vi "main 0.6.vi"() -> ()   [LabVIEW 2015]
uses:
  subvi/PHOIBOS/DEFINITIONS/DEF_dev_state.ctl
  subvi/PHOIBOS/DEFINITIONS/DEF_dev_type.ctl
  <vilib>/Utility/file.llb/Write Delimited Spreadsheet (DBL).vi
  subvi/Newport ESP301/Newport ESP301.lvlib
  subvi/sp_manip.llb/sp_manip_lib.lvlib
  subvi/sp_manip.llb/tcp_gateway.lvlib
panel:
  out "RunNumber":u16=4
  out "# elements in queue":i32
  out "sum":dbl=3886353.0
  out "cam_fps":dbl(slide)=19.67681433793903 caption="FPS" scale=0.1..50.0
  out "max value":u32=54
  out "Intensity Graph":dbl[][](graph)
  out "ESP_con?":bool=TRUE caption="ESP301"
  out "phoib_con?":bool caption="PHOIBOS"
  out "manip_con?":bool caption="manipulator"
  out "cam_con?":bool caption="camera"
  in  "main_close":bool
  in  "Tab Control":T1(tab)
  in  "cam_avg":u32=20
  in  "ESP_delta":dbl caption="relative [mm]"
  in  "ESP_-":bool
  in  "ESP_+":bool
  in  "ESP_go":bool
  in  "ESP_dest_t":dbl caption="Delay [fs]"
  in  "ESP_dest":dbl=33.3075 caption="Position [mm]"
  in  "ESP_set_t0":bool
  in  "phoib_I_6s":dbl=3200.0
  in  "phoib_I_5s":dbl=1400.0
  in  "phoib_I_4s":dbl=4.2
  in  "phoib_I_3s":dbl
  in  "phoib_I_2s":dbl=35.0
  in  "phoib_I_1s":dbl=21.9
  in  "phoib_standby":bool
  in  "phoib_set":bool
  out "phoib_I_6":dbl caption="Screen Voltage"
  out "phoib_I_5":dbl caption="Detctor Voltage"
  out "phoib_I_4":dbl caption="Work Function"
  out "phoib_I_3":dbl caption="Coil Current"
  out "phoib_I_2":dbl caption="Pass Energy"
  out "phoib_I_1":dbl caption="Kinetic Energy"
  out "Saved Positions":string[][](table)=[["ertwertwert", "-2.299945", "-2.030214", "38.900024", "50.000762", "0.000887", "-97.998082"], ["uztgugt", "-14.999451", "-13.638894", "442.380066", "13.998380", "-1.893758", "-76.305838"], ["asdf", "-14.999451", "-13.638894", "442.380066", "13.998380", "-1.893758", "-76.305838"], ["test3", "-14.999451", "-13.638894", "441.380066", "13.998380", "-1.893758", "-76.305838"]]
  in  "Save Pos":bool
  in  "Load":bool
  in  "Delete":bool
  in  "ManipRel":dbl=1.0
  in  "ManipRel +":bool
  in  "ManipRel -":bool
  in  "manip.rel.select":enum32{"x", "y", "z", "polar", "tilt", "azimut"}(radio)=enum."polar"
  in  "Move Abs":bool
  in  "stop manip":bool
  in  "dest":dbl[](array[numeric])=[0.007141549166819264, -0.009888298846365134, 431.30615234375, 89.00040512814502, 1.109125024699864, -227.9162918846475] caption="destinations" format="%#.5g"
  out "names":string[](array[string])=["x", "y", "z", "polar", "tilt", "azimut"]
  out "pos":dbl[](array[numeric])=[0.007141549166819264, -0.009888298846365134, 431.30615234375, 89.00040512814502, 1.109125024699864, -227.9162918846475] caption="positions" format="%.5f"
  in  "Mode":T2(ring)=enum."WideAngleMode"
  in  "VoltageRange":enum16{"3.5kV", "1.5kV", "400V", "100V", "10V"}(ring)=enum."400V"
  out "ESP_pos":dbl=33.3075 caption="Position"
  out "ESP_delay":dbl caption="Delay"
  out "ESP_t0":dbl=33.3075 caption="Time Zero @"
  out "phoib_I_7":dbl caption="Conversion Voltage"
  in  "phoib_I_7s":dbl
  in  "phoib_I_8s":dbl
  in  "phoib_I_9s":dbl
  out "phoib_I_8":dbl caption="FD1"
  out "phoib_I_9":dbl caption="FD2"
  out "electronics temp [°C]":i32=30
  out "CCD temp [°C]":i32=-13
  in  "gain":bool
  in  "exposure [ms]":u32=20
  in  "binning":u16(ring)=2 items=["X 1", "X 2", "X 4", "X 8"]
  in  "cam_dark?":bool caption="subtract dark?"
  in  "cam_dark":bool
  in  "cam_dark#":u32 max=1000
  in  "cam_burst":bool
  in  "cam_burstnr":u32 max=100000
  out "cam_burst_progress":i32(slide) scale=0.0..10.0
  out "Motion Done":bool
  in  "delscan_picspstep":u16=1 caption="pics/step" min=1 step=1
  in  "delscan_abort":bool
  out "delscan_progress":u32(slide) scale=0.0..20.0
  in  "delscan_go":bool
  out "delscan_pos":dbl caption="current delay [fs]"
  in  "delscan_end":dbl caption="end [fs]"
  in  "delscan_stepsize":dbl caption="stepsize [fs]"
  in  "delscan_start":dbl caption="start [fs]"
  in  "comment":string
  out "opti_frames":dbl=25.0 caption="#steps_opti"
  out "opti_current_frame":i32=25
  out "Measurement Progress":u8(slide) scale=0.0..100.0
  out "Camera Aquisition":u8(slide) scale=0.0..100.0
  in  "Optimize":bool
  in  "OptiStepSize":dbl=-1.0 caption="Step Size"
  in  "OptiRange":dbl=25.0 caption="Range"
  in  "meas_axis":string(combo)="tilt" caption="Axis"
  in  "meas_avg":i32=60 caption="Frames2Average"
  in  "OptiCancel":bool
  out "#steps_opti":dbl=25.0
  out "current_step_opti":i32=25
  out "ETA":string
  in  "BasePath":path=path "Z:/PESdata"
  in  "Path":path=path "Z:/software/ManipulatorControl/save.txt"
  in  "ROI Bottom":i32=32
  in  "ROI Top":i32=1
  in  "ROI Right":i32=40
  in  "ROI Left":i32=1
  in  "ESP Axis":i32=1 min=1 max=3
  in  "manip_init":bool
  in  "manip_release":bool
  in  "phoib_init":bool
  in  "phoib_release":bool
  in  "ESP_init":bool
  in  "ESP_release":bool
  in  "ESP301 VISA":refnum<visa-resource-name>="COM8"
  in  "cam_boardnr":i32
  in  "cam_init":bool
  in  "cam_release":bool
  out "error out":errorcluster
  out "error out 2":errorcluster
  out "state":T3 items=["Off"=-1, "Standby"=0, "On"=1]
  # "step _ of _"
  # "step _ of _"
  # "manip"
  # "phoib"
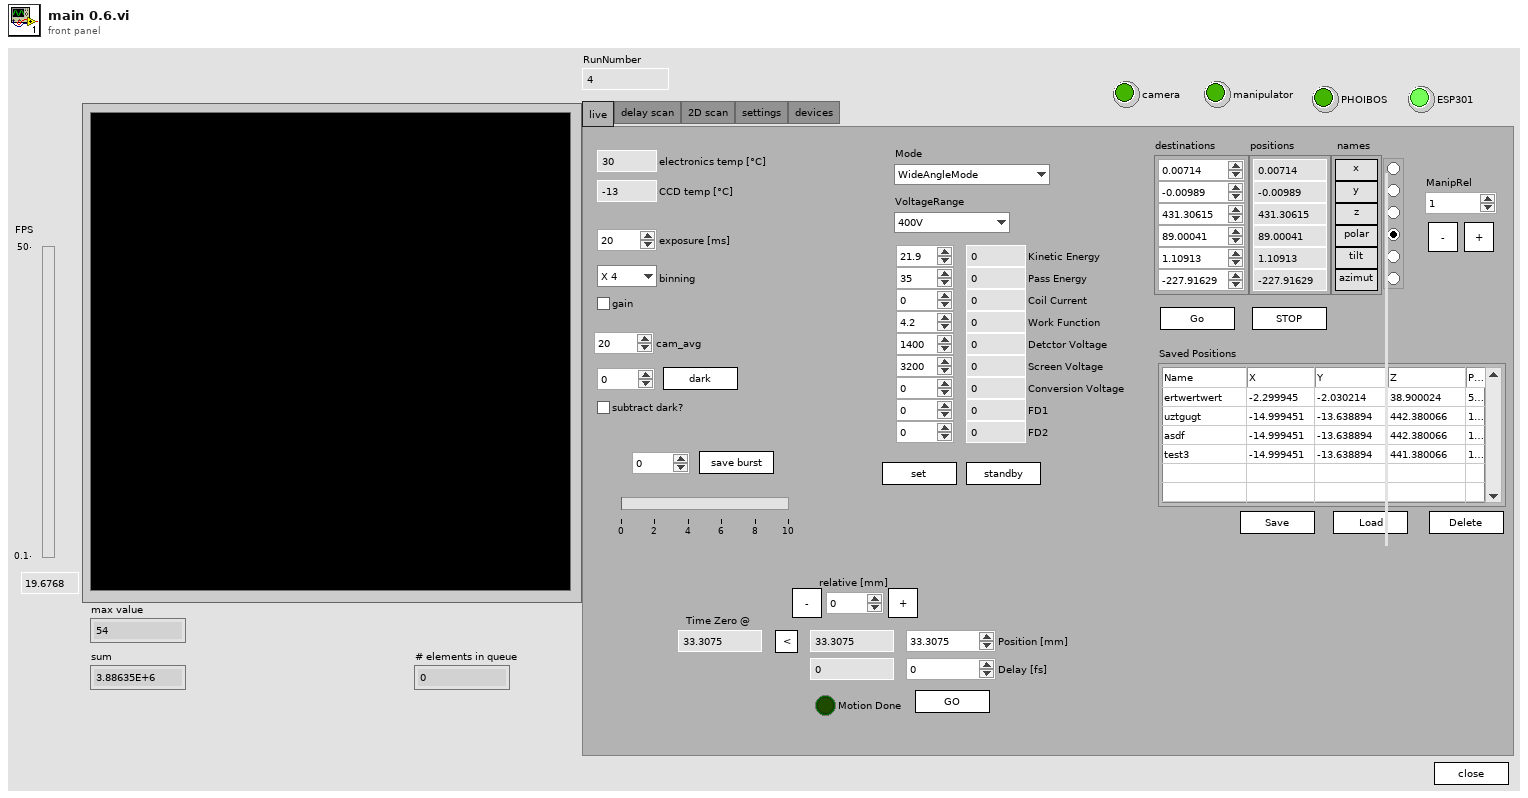
[diagram p1: front panel]
types:
  T1 = enum32{"live", "delay scan", "2D scan", "settings", "devices"}
  T2 = enum16{"HighMagnification", "MediumMagnification", "LowMagnification", "HighAngularDispersion", "MediumAngularDispersion", "LowAngularDispersion", "WideAngleMode", "LargeArea", "MediumArea", "SmallArea", "HighMagnification2", "SmallArea2", "ImagingMode"}
  T3 = typedef "DEF_dev_state.ctl" = i32
  T4 = enum16{"open", "replace", "create", "open or create", "replace or create", "replace or create with confirmation"}
  T5 = cluster{"Camera type":u32, "Operating mode\nHP & QE / HS & DiCam Pro ":u32, "Frame trigger \n(High Performance and QE only)":u16, "Sequence trigger":u16, "Low Light\n(QE only)":bool, "Gain":bool, "Horzontal\nbinning":u16, "Vertical\nbinning ":u16, "ROI Left":i32, "ROI Right":i32, "ROI Top":i32, "ROI Bottom":i32}
  T6 = cluster{"Axis_Name":string, "Axis_Type":string, "Axis_Position":dbl, "continous":bool, "moving":bool}[]
  T7 = cluster{"Axis_Name":string, "Axis_Type":string, "Axis_Position":dbl, "continous":bool, "moving":bool}
  T8 = typedef "DEF_dev_type.ctl" = enum32{"devA (analyzer)", "devD (detector)"}
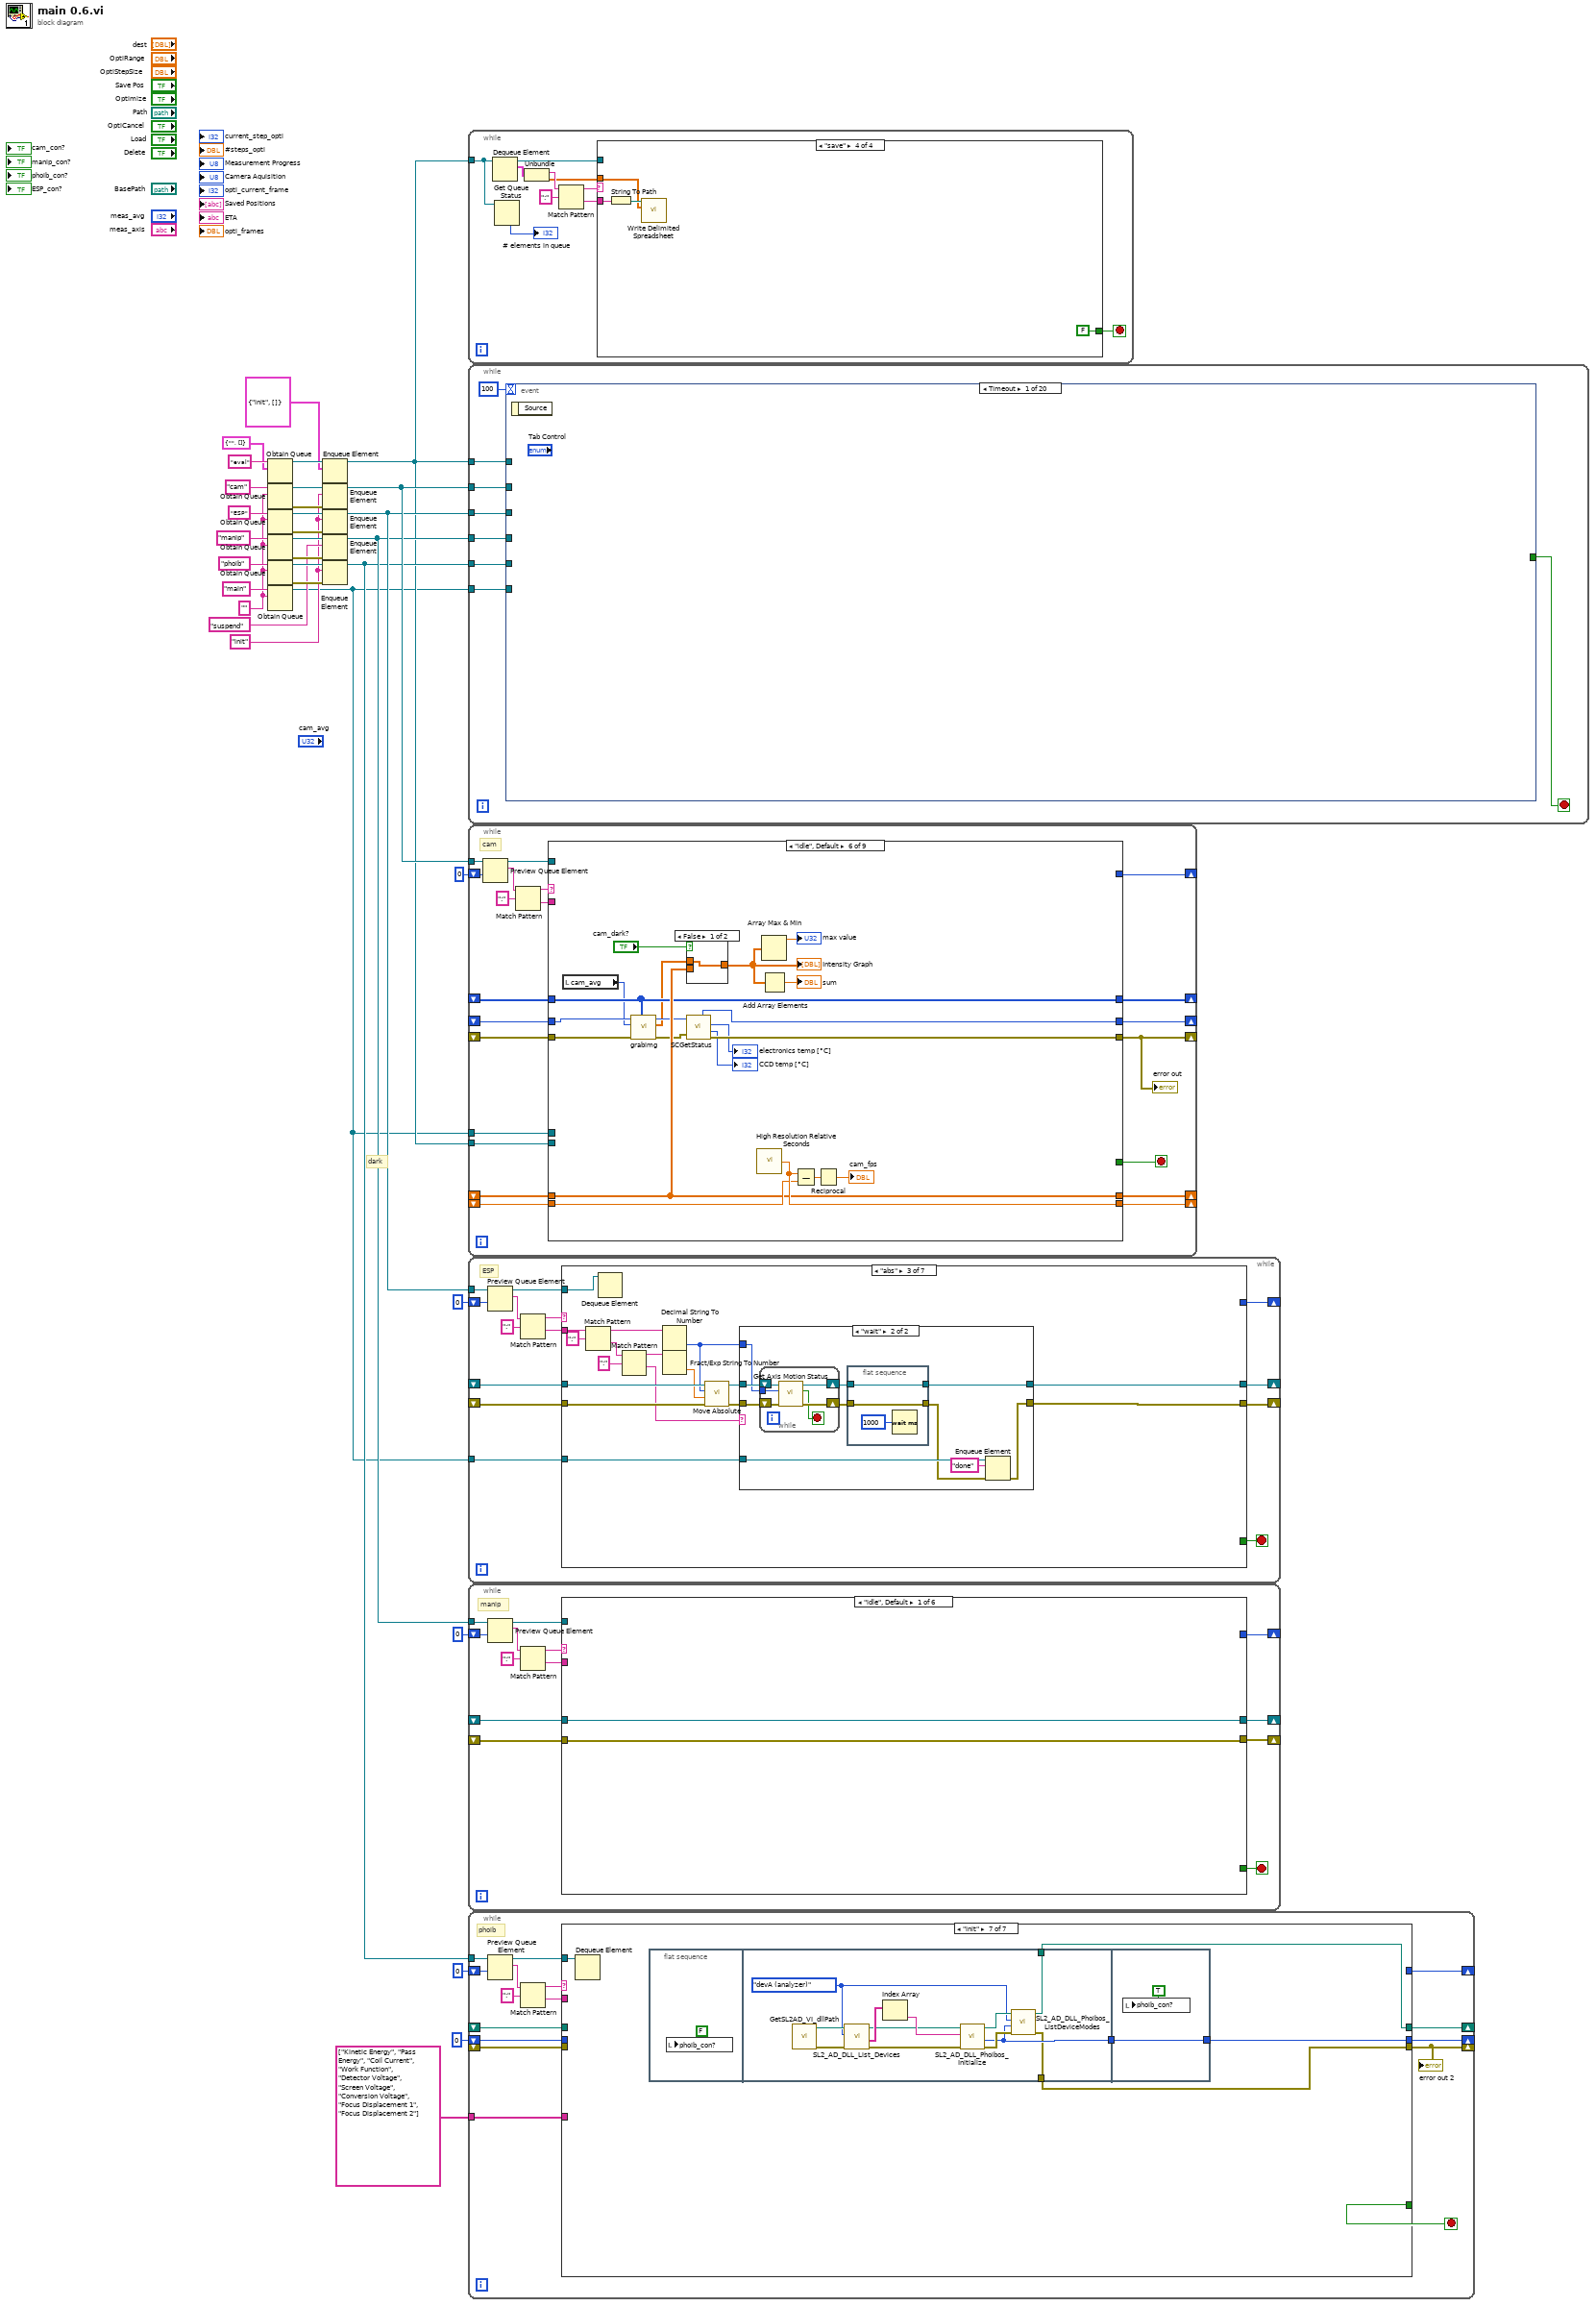
[diagram p0: block diagram]
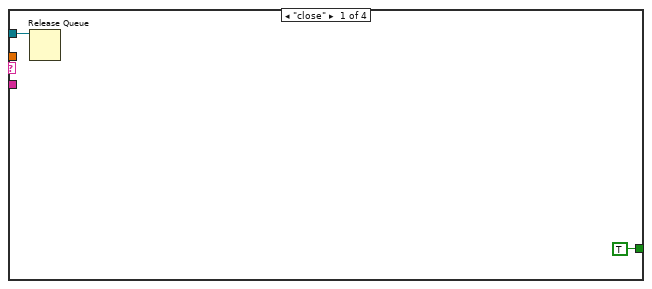
[diagram p2: hidden frame]
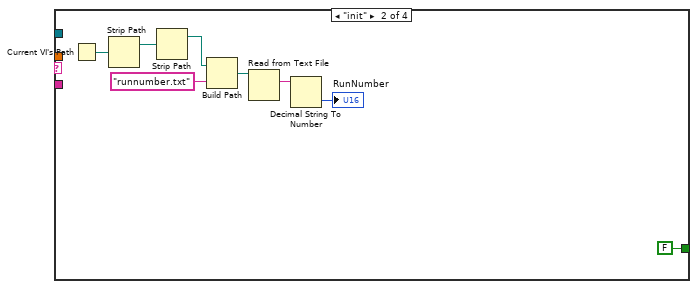
[diagram p3: hidden frame]
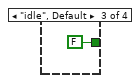
[diagram p4: hidden frame]
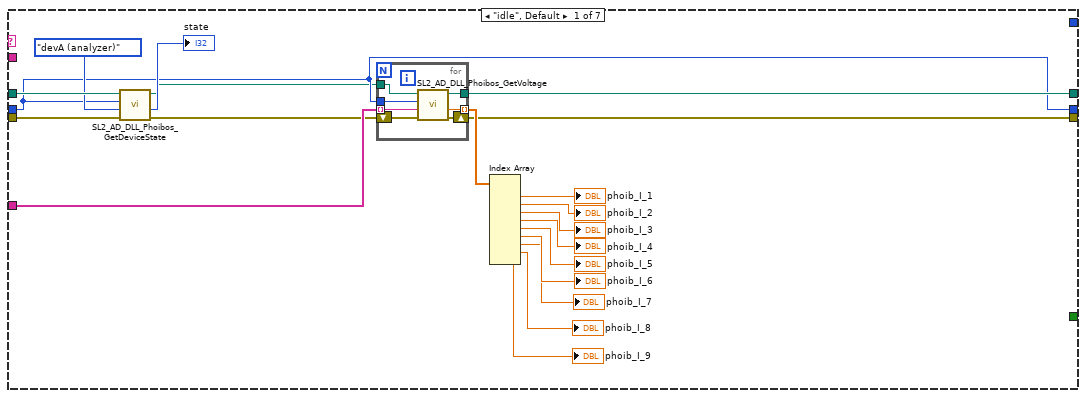
[diagram p5: hidden frame]
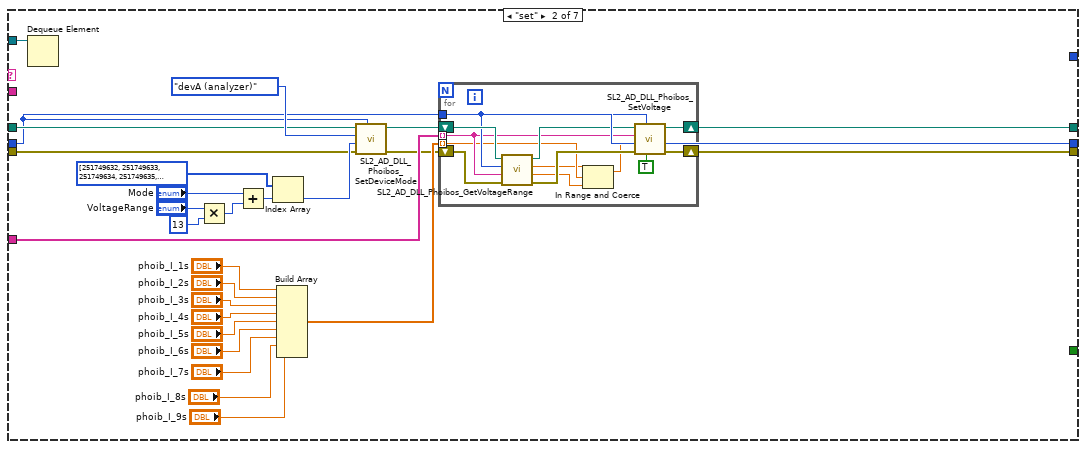
[diagram p6: hidden frame]
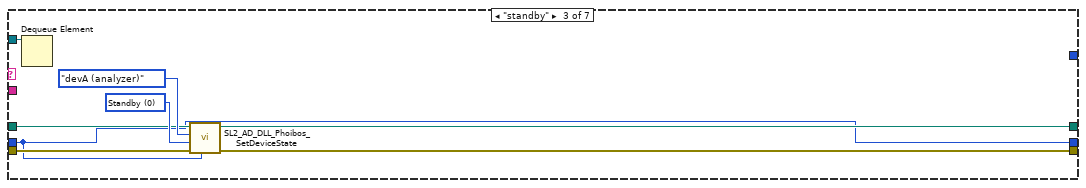
[diagram p7: hidden frame]
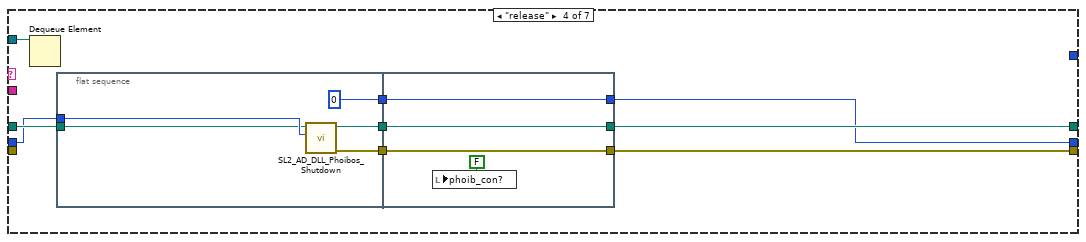
[diagram p8: hidden frame]
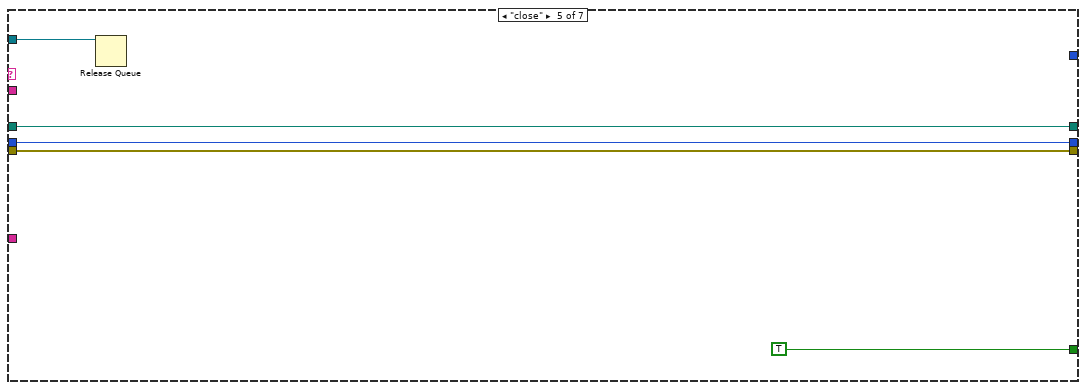
[diagram p9: hidden frame]
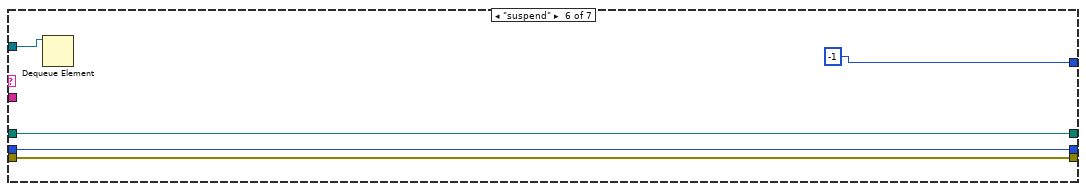
[diagram p10: hidden frame]
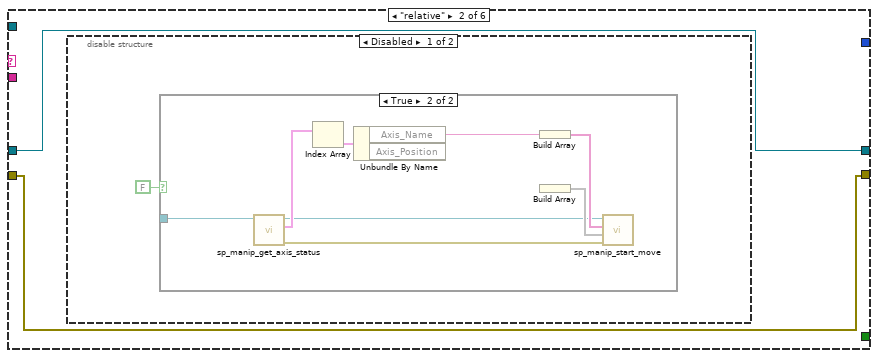
[diagram p11: hidden frame]
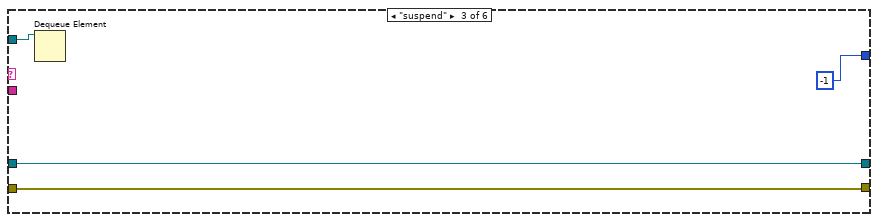
[diagram p14: hidden frame]
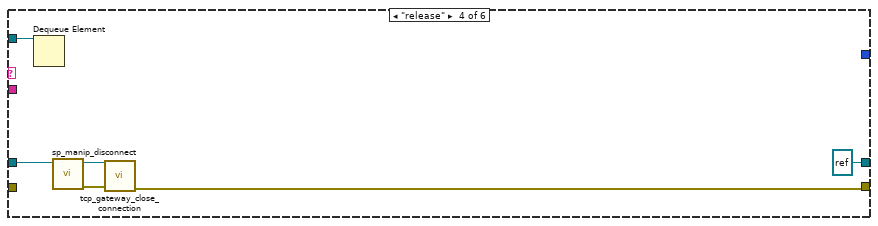
[diagram p15: hidden frame]
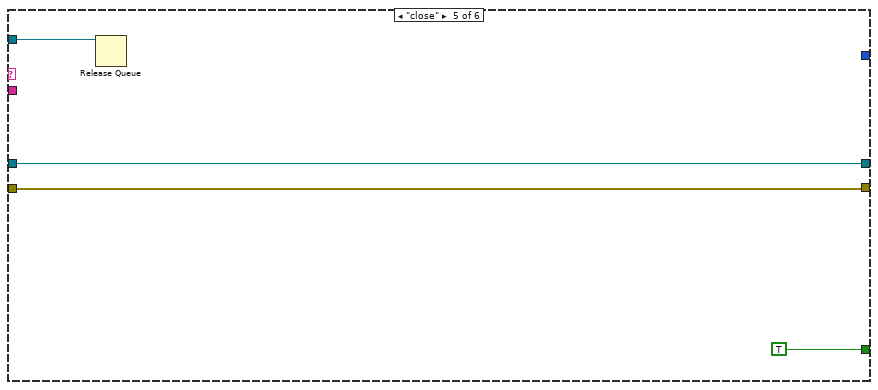
[diagram p16: hidden frame]
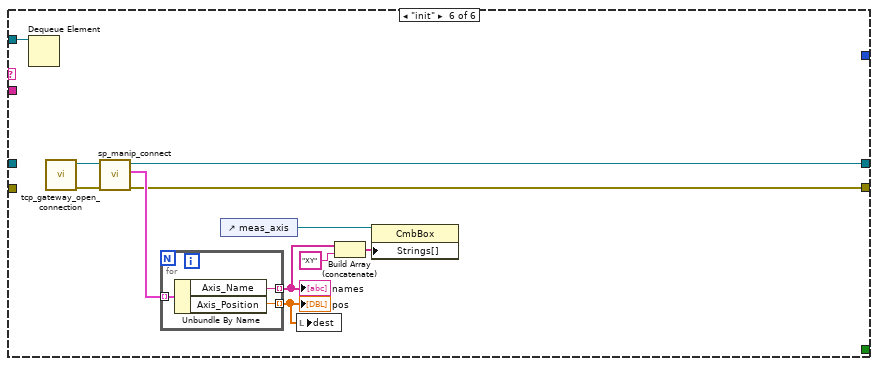
[diagram p17: hidden frame]
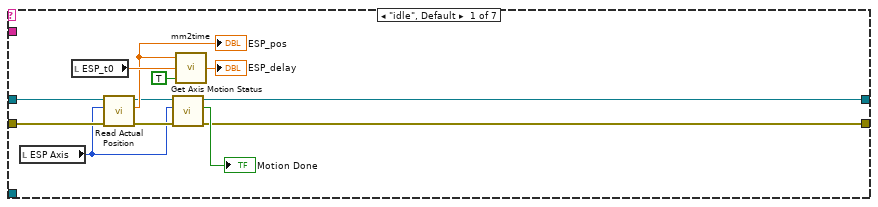
[diagram p18: hidden frame]
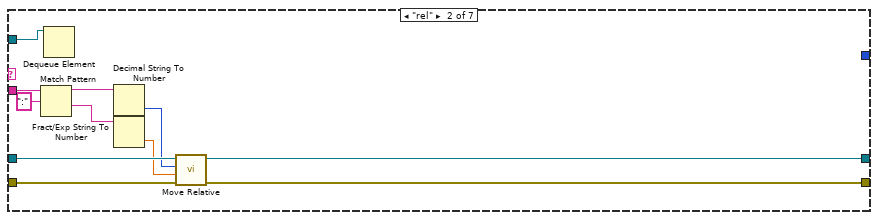
[diagram p19: hidden frame]
diagram:
  w3 = "init" ("name (unnamed)")
  w8 = "" ("name (unnamed)")
  # "dark"
  n1 = Obtain Queue(name (unnamed)="eval", element data type=cluster{string, dbl[][]} {"", []}) -> (queue out=w6:refnum<queue>)  [unwired: 3 in, 2 out]
  n2 = Obtain Queue(name (unnamed)="cam", element data type=w8) -> (queue out=w31:refnum<queue>, error out=w30:errorcluster)  [unwired: 3 in, 1 out]
  n3 = Obtain Queue(name (unnamed)="ESP", element data type=w8) -> (queue out=w27:refnum<queue>, error out=w28:errorcluster)  [unwired: 3 in, 1 out]
  n4 = Obtain Queue(name (unnamed)="manip", element data type=w8) -> (queue out=w24:refnum<queue>, error out=w23:errorcluster)  [unwired: 3 in, 1 out]
  n5 = Obtain Queue(name (unnamed)="phoib", element data type=w8) -> (queue out=w21:refnum<queue>, error out=w22:errorcluster)  [unwired: 3 in, 1 out]
  n6 = Obtain Queue(name (unnamed)="main", element data type=w8) -> (queue out=w1:refnum<queue>)  [unwired: 3 in, 2 out]
  n7 = Enqueue Element(queue=w6, element=cluster{string, dbl[][]} {"init", []}) -> (queue out=w5:refnum<queue>)  [unwired: 2 in, 2 out]
  n8 = Enqueue Element(queue=w31, element=w3, error in (no error)=w30) -> (queue out=w29:refnum<queue>)  [unwired: 1 in, 2 out]
  n9 = Enqueue Element(queue=w27, element=w3, error in (no error)=w28) -> (queue out=w18:refnum<queue>)  [unwired: 1 in, 2 out]
  n10 = Enqueue Element(queue=w24, element="suspend" ("name (unnamed)"), error in (no error)=w23) -> (queue out=w17:refnum<queue>)  [unwired: 1 in, 2 out]
  n11 = Enqueue Element(queue=w21, element=w3, error in (no error)=w22) -> (queue out=w16:refnum<queue>)  [unwired: 1 in, 2 out]
  n12 = while {
    tunnel: w5 -> [w34]
    stop <- w35 stop-if-true
    n13 = Dequeue Element(queue=w34) -> (queue out=w40:refnum<queue>, element=w39:cluster{string, dbl[][]})  [unwired: 2 in, 2 out]
    n14 = Get Queue Status(queue=w34) -> (# elements in queue=→"# elements in queue":i32)  [unwired: 2 in, 7 out]
    n15 = Unbundle(w39) -> (w38:string, w37:dbl[][])
    n16 = Match Pattern(string=w38, regular expression=":") -> (before substring=w41:string, after substring=w36:string)  [unwired: 1 in, 2 out]
    n17 = case shown="\"save\"" w41 {
      tunnel: w40 -> [w44 _ _ _]
      tunnel: w37 -> [_ _ _ w55]
      tunnel: w36 -> [_ _ _ w57]
      tunnel: [TRUE FALSE FALSE FALSE] -> w35
      frame "close" {
        n18 = Release Queue(queue=w44) -> ()  [unwired: 2 in, 3 out]
      }
      frame "init" {
        n19 = Current VI's Path() -> (path=w51:path)
        n20 = Strip Path(path=w51) -> (stripped path=w46:path)  [unwired: 1 out]
        n21 = Strip Path(path=w46) -> (stripped path=w45:path)  [unwired: 1 out]
        n22 = Build Path(base path=w45, name or relative path="runnumber.txt") -> (appended path=w49:path)
        n23 = Read from Text File(file (use dialog)=w49) -> (text=w48:string)  [unwired: 3 in, 3 out]
        n24 = Decimal String To Number(string=w48) -> (number=→"RunNumber":i32)  [unwired: 2 in, 1 out]
      }
      frame "idle", Default {
      }
      frame "save" {
        n25 = String To Path(string=w57) -> (path=w56:path)
        n26 = call-poly <vilib>:"Write Delimited Spreadsheet.vi"("file path (dialog if empty)"=w56, "2D data"=w55) -> ()  [unwired: 12 in, 2 out]
      }
    }
  }
  n27 = while {
    tunnel: w29 -> [w63]
    tunnel: w18 -> [w62]
    tunnel: w17 -> [w61]
    tunnel: w16 -> [w60]
    tunnel: w1 -> [w59]
    tunnel: w5 -> [w58]
    stop <- w65 stop-if-true
    n28 = event shown="[0] Timeout" {
      selector: _ -> [_ _ _ _ _ _ _ _ _ _ _ _ _ _ _ _ _ _ _ _]
      dyn-events: _ -> [_ _ _ _ _ _ _ _ _ _ _ _ _ _ _ _ _ _ _ _]
      timeout: 100 -> [_ _ _ _ _ _ _ _ _ _ _ _ _ _ _ _ _ _ _ _]
      tunnel: [_ TRUE _ _ _ _ _ _ _ _ _ _ _ _ _ _ _ _ _ _] -> w65
      tunnel: w63 -> [_ w78 w81 _ _ _ _ _ w107 w109 w110 _ _ _ _ _ _ _ _ w202]
      tunnel: w62 -> [_ w77 _ w85 _ _ _ _ _ _ _ _ _ _ w156 _ w168 _ _ w204]
      tunnel: w61 -> [_ w76 _ _ w91 _ _ _ _ _ _ _ _ _ _ _ _ _ _ _]
      tunnel: w60 -> [_ w75 _ _ _ w97 w103 w104 _ _ _ _ _ _ _ _ _ _ _ _]
      tunnel: w59 -> [_ w68 _ _ _ _ _ _ _ _ _ _ _ _ _ _ _ _ _ w203]
      tunnel: w58 -> [_ w67 _ _ _ _ _ _ _ _ _ _ _ _ _ _ _ _ _ _]
      event Timeout {
        n29 = event-data() -> ()  [unwired: 1 in, 1 out]
      }
      event "main_close": Value Change {
        w69 = "close" ("element")
        w74 = "release" ("element")
        n30 = event-data() -> ()  [unwired: 1 in, 1 out]
        n31 = Enqueue Element(queue=w78, element=w74) -> (queue out=w73:refnum<queue>)  [unwired: 2 in, 2 out]
        n32 = Enqueue Element(queue=w77, element=w74) -> (queue out=w72:refnum<queue>)  [unwired: 2 in, 2 out]
        n33 = Enqueue Element(queue=w76, element=w74) -> (queue out=w71:refnum<queue>)  [unwired: 2 in, 2 out]
        n34 = Enqueue Element(queue=w75, element=w74) -> (queue out=w70:refnum<queue>)  [unwired: 2 in, 2 out]
        n35 = Release Queue(queue=w68) -> ()  [unwired: 2 in, 3 out]
        n36 = Enqueue Element(queue=w67, element=cluster{string, dbl[][]} {"close", []}) -> ()  [unwired: 2 in, 3 out]
        n37 = Enqueue Element(queue=w73, element=w69) -> ()  [unwired: 2 in, 3 out]
        n38 = Enqueue Element(queue=w72, element=w69) -> ()  [unwired: 2 in, 3 out]
        n39 = Enqueue Element(queue=w71, element=w69) -> ()  [unwired: 2 in, 3 out]
        n40 = Enqueue Element(queue=w70, element=w69) -> ()  [unwired: 2 in, 3 out]
      }
      event "cam_release", "cam_init": Value Change {
        n41 = event-data() -> ()  [unwired: 1 in, 2 out]
        n42 = Select(t="init" ("name (unnamed)"), s="cam_init", f="release" ("name (unnamed)")) -> (s? t:f=w80:string)
        n43 = Enqueue Element(queue=w81, element=w80) -> ()  [unwired: 2 in, 3 out]
      }
      event "ESP_release", "ESP_init": Value Change {
        n44 = event-data() -> ()  [unwired: 1 in, 2 out]
        n45 = Select(t="init" ("name (unnamed)"), s="ESP_init", f="release" ("name (unnamed)")) -> (s? t:f=w89:string)
        n46 = Enqueue Element(queue=w85, element=w89) -> ()  [unwired: 2 in, 3 out]
      }
      event "manip_init", "manip_release": Value Change {
        n47 = event-data() -> ()  [unwired: 1 in, 2 out]
        n48 = Flush Queue(queue=w91) -> (queue out=w90:refnum<queue>)  [unwired: 1 in, 2 out]
        n49 = Select(t="init" ("name (unnamed)"), s="manip_init", f="release" ("name (unnamed)")) -> (s? t:f=w93:string)
        n50 = Enqueue Element(queue=w90, element=w93) -> ()  [unwired: 2 in, 3 out]
      }
      event "phoib_release", "phoib_init": Value Change {
        n51 = event-data() -> ()  [unwired: 1 in, 2 out]
        n52 = Flush Queue(queue=w97) -> (queue out=w96:refnum<queue>)  [unwired: 1 in, 2 out]
        n53 = Select(t="init" ("name (unnamed)"), s="phoib_init", f="release" ("name (unnamed)")) -> (s? t:f=w99:string)
        n54 = Enqueue Element(queue=w96, element=w99) -> ()  [unwired: 2 in, 3 out]
      }
      event "phoib_standby": Value Change {
        n55 = event-data() -> ()  [unwired: 1 in, 2 out]
        n56 = Enqueue Element(queue=w103, element="standby") -> ()  [unwired: 2 in, 3 out]
      }
      event "phoib_set": Value Change {
        n57 = event-data() -> ()  [unwired: 1 in, 2 out]
        n58 = Enqueue Element(queue=w104, element="set") -> ()  [unwired: 2 in, 3 out]
      }
      event "cam_dark": Value Change {
        n59 = event-data() -> ()  [unwired: 1 in, 2 out]
        n60 = Enqueue Element(queue=w107, element="dark") -> ()  [unwired: 2 in, 3 out]
      }
      event "ROI Left", "ROI Right", "ROI Top", "ROI Bottom", "exposure [ms]", "binning", "gain": Value Change {
        n61 = event-data() -> ()  [unwired: 1 in, 1 out]
        n62 = Enqueue Element(queue=w109, element="set") -> ()  [unwired: 2 in, 3 out]
      }
      event "cam_burst": Value Change {
        n63 = event-data() -> ()  [unwired: 1 in, 1 out]
        n64 = local read "BasePath"() -> (w114:path)
        n65 = call "File Dialog"("start path"=w114) -> ("selected path"=w112:path, "cancelled"=w113:bool, "error out"=w111:errorcluster)  [unwired: 11 in, 1 out]
        n66 = case shown="False" w113 {
          tunnel: w112 -> [w138 _]
          tunnel: w111 -> [_ _]
          tunnel: w110 -> [w145 _]
          frame False {
            w133 = "\r"
            w132 = "\t"
            n67 = local read "exposure [ms]"() -> (w125:u32)
            n68 = local read "binning"() -> (w123:u16)
            n69 = local read "gain"() -> (w124:bool)
            n70 = Boolean To (0,1)(Boolean=w124) -> (0, 1=w122:i16)
            n71 = Number To Decimal String(number=w125) -> (decimal integer string=w120:string)  [unwired: 1 in]
            n72 = Number To Decimal String(number=w122) -> (decimal integer string=w118:string)  [unwired: 1 in]
            n73 = Number To Decimal String(number=w123) -> (decimal integer string=w116:string)  [unwired: 1 in]
            n74 = Get Date/Time In Seconds() -> (seconds since 1Jan1904=w136:timestamp)
            n75 = Format Date/Time String(time format string (%c)="%Y.%m.%d-%H.%M.%S", seconds (now)=w136) -> (date/time string=w135:string)  [unwired: 1 in]
            n76 = Concatenate Strings("Exposure:", w132, w120, w133, "Gain:", w132, w118, w133, "binning", w132, w116, w133) -> (w126:string)
            n77 = Build Path(base path=w138, name or relative path=w135) -> (appended path=w134:path)
            n78 = Create Folder(path (use dialog)=w134) -> (created path=w115:path)  [unwired: 2 in, 2 out]
            n79 = Build Path(base path=w115, name or relative path="info.txt") -> (appended path=w130:path)
            n80 = Number To Decimal String(number="cam_burstnr") -> (decimal integer string=w142:string)  [unwired: 1 in]
            n81 = Path To String(path=w115) -> (string=w140:string)
            n82 = Open/Create/Replace File(file path (use dialog)=w130, operation (0:open)=T4."replace or create") -> (refnum out=w128:refnum<file>)  [unwired: 4 in, 2 out]
            n83 = Write to Text File(file (use dialog)=w128, text=w126) -> (refnum out=w127:refnum<file>)  [unwired: 2 in, 2 out]
            n84 = Close File(refnum=w127) -> ()  [unwired: 1 in, 2 out]
            n85 = Concatenate Strings("burst:" ("string"), w142, ":" ("string"), w140) -> (w139:string)
            n86 = Enqueue Element(queue=w145, element=w139) -> ()  [unwired: 2 in, 3 out]
          }
          frame True {
          }
        }
      }
      event "Move Abs": Value Change {
        n87 = event-data() -> ()  [unwired: 1 in, 1 out]
      }
      event "ManipRel +", "ManipRel -": Value Change {
        n88 = event-data() -> ()  [unwired: 1 in, 2 out]
        n89 = Negate(x="ManipRel") -> (-x=w147:dbl)
        n90 = Select(t=w147, s="ManipRel -", f="ManipRel") -> ()  [unwired: 1 out]
      }
      event "stop manip": Value Change {
        n91 = event-data() -> ()  [unwired: 1 in, 1 out]
      }
      event "ESP_go": Value Change {
        w150 = ":" ("string")
        n92 = event-data() -> ()  [unwired: 1 in, 1 out]
        n93 = local read "ESP Axis"() -> (w149:i32)
        n94 = Number To Decimal String(number=w149) -> (decimal integer string=w152:string)  [unwired: 1 in]
        n95 = Number To Fractional String(number="ESP_dest") -> (F-format string=w151:string)  [unwired: 3 in]
        n96 = Concatenate Strings("abs:" ("string"), w152, w150, w151, w150) -> (w155:string)
        n97 = Enqueue Element(queue=w156, element=w155) -> ()  [unwired: 2 in, 3 out]
      }
      event "ESP_set_t0": Value Change {
        n98 = event-data() -> ()  [unwired: 1 in, 1 out]
        n99 = Current VI's Path() -> (path=w162:path)
        n100 = Strip Path(path=w162) -> (stripped path=w158:path)  [unwired: 1 out]
        n101 = Strip Path(path=w158) -> (stripped path=w157:path)  [unwired: 1 out]
        n102 = local read "ESP_pos"() -> (w160:dbl)
        "ESP_t0" <- w160
        n103 = Number To Fractional String(number=w160) -> (F-format string=w159:string)  [unwired: 3 in]
        n104 = Build Path(base path=w157, name or relative path="t0.txt") -> (appended path=w161:path)
        n105 = Write to Text File(file (use dialog)=w161, text=w159) -> ()  [unwired: 2 in, 3 out]
      }
      event "ESP_+", "ESP_-": Value Change {
        n106 = event-data() -> ()  [unwired: 1 in, 6 out]
        n107 = Negate(x="ESP_delta") -> (-x=w171:dbl)
        n108 = Select(t="ESP_delta", s="ESP_+", f=w171) -> (s? t:f=w169:dbl)
        n109 = Number To Decimal String(number="ESP Axis") -> (decimal integer string=w166:string)  [unwired: 1 in]
        n110 = Number To Fractional String(number=w169) -> (F-format string=w164:string)  [unwired: 3 in]
        n111 = Concatenate Strings("rel:" ("string"), w166, ":" ("string"), w164) -> (w174:string)
        n112 = Enqueue Element(queue=w168, element=w174) -> ()  [unwired: 2 in, 3 out]
      }
      event "ESP_dest": Value Change {
        n113 = event-data() -> ()  [unwired: 1 in, 6 out]
        n114 = local read "ESP_dest"() -> (w178:dbl)
        n115 = local read "ESP_t0"() -> (w177:dbl)
        n116 = call "mm2time.vi"("fs?"=TRUE ("fs[1]/ps[0]"), "Offset (mm)"=w177, "distance (mm)"=w178) -> ("time in fs/ps seconds"=w175:dbl)
        n117 = local write "ESP_dest_t"(w175) -> ()
      }
      event "ESP_dest_t": Value Change {
        n118 = event-data() -> ()  [unwired: 1 in, 1 out]
        n119 = local read "ESP_t0"() -> (w181:dbl)
        n120 = call "time2mm.vi"("fs[1]/ps[0]"=TRUE, "Offset (mm)"=w181, "time"="ESP_dest_t") -> ("position (mm)"=w179:dbl)
        n121 = local write "ESP_dest"(w179) -> ()
      }
      event "delscan_go": Value Change {
        n122 = event-data() -> ()  [unwired: 1 in, 1 out]
        n123 = local read "RunNumber"() -> (w201:u16)
        n124 = local read "BasePath"() -> (w200:path)
        n125 = Increment(x=w201) -> (x+1=w184:u16)
        n126 = call "create_opti_path.vi"("N"="delscan_picspstep", "RunNumber"=w184, "comment"="comment", "base path"=w200) -> ("Path"=w197:path)
        n127 = local write "RunNumber"(w184) -> ()
        n128 = Number To Decimal String(number=w184) -> (decimal integer string=w183:string)  [unwired: 1 in]
        n129 = Subtract(x="delscan_end", y="delscan_start") -> (x-y=w194:dbl)
        n130 = Divide(x=w194, y="delscan_stepsize") -> (x/y=w192:dbl)
        n131 = property on="delscan_progress" class="Slide (strict)"("Scale.Maximum"=w192) -> ()  [unwired: 2 in, 2 out]
        n132 = Current VI's Path() -> (path=w191:path)
        n133 = while {
          tunnel: "delscan_stepsize" -> [w234]
          tunnel: "delscan_start" -> [w232]
          tunnel: "delscan_end" -> [w231]
          tunnel: w204 -> [w223]
          tunnel: w203 -> [w205]
          tunnel: w202 -> [w217]
          tunnel: "delscan_picspstep" -> [w215]
          tunnel: w197 -> [w214]
          i -> [w218]
          stop <- w211 stop-if-true
          w210 = ":" ("string")
          n134 = Multiply(x=w234, y=w218) -> (x*y=w233:dbl)
          n135 = Add(x=w232, y=w233) -> (x+y=w225:dbl)
          n136 = local read "ESP_t0"() -> (w226:dbl)
          n137 = Greater?(x=w225, y=w231) -> (0:w213:bool)
          n138 = local read "ESP Axis"() -> (w224:i32)
          n139 = call "time2mm.vi"("fs[1]/ps[0]"=TRUE, "Offset (mm)"=w226, "time"=w225) -> ("position (mm)"=w222:dbl)
          "delscan_pos" <- w222
          n140 = Number To Decimal String(number=w224) -> (decimal integer string=w228:string)  [unwired: 1 in]
          n141 = Number To Fractional String(number=w222) -> (F-format string=w216:string)  [unwired: 3 in]
          n142 = Concatenate Strings("abs:" ("string"), w228, w210, w216, w210, "wait" ("string")) -> (w230:string)
          n143 = Enqueue Element(queue=w223, element=w230) -> (error out=w221:errorcluster)  [unwired: 2 in, 2 out]
          n144 = Dequeue Element(queue=w205, timeout in ms (-1)=10000, error in (no error)=w221) -> (element=w220:string)  [unwired: 3 out]
          n145 = Equal?(x=w220, y="done") -> (x = y?=w209:bool)
          n146 = Not(x=w209) -> (.not. x?=w208:bool)
          n147 = Compound Arithmetic op=OR("delscan_abort", w213, w208) -> (w211:bool)
          n148 = case shown="True" w209 {
            tunnel: w217 -> [_ w250]
            tunnel: w216 -> [_ w246]
            tunnel: w215 -> [_ w241]
            tunnel: w214 -> [_ w240]
            tunnel: w205 -> [_ w237]
            frame False {
              n149 = One Button Dialog(message="esp error") -> ()  [unwired: 1 in, 1 out]
            }
            frame True {
              n150 = Build Path(base path=w240, name or relative path=w246) -> (appended path=w244:path)
              n151 = Number To Decimal String(number=w241) -> (decimal integer string=w247:string)  [unwired: 1 in]
              n152 = Path To String(path=w244) -> (string=w243:string)
              n153 = Concatenate Strings(w243, ".tsv" ("string")) -> (w245:string)
              n154 = Concatenate Strings("snap:" ("element"), w247, ":" ("string"), w245) -> (w249:string)
              n155 = Enqueue Element(queue=w250, element=w249) -> (error out=w236:errorcluster)  [unwired: 2 in, 2 out]
              n156 = Dequeue Element(queue=w237, timeout in ms (-1)=30000, error in (no error)=w236) -> ()  [unwired: 4 out]
            }
          }
          "delscan_progress" <- w218
        }
        n157 = Strip Path(path=w191) -> (stripped path=w190:path)  [unwired: 1 out]
        n158 = Strip Path(path=w190) -> (stripped path=w189:path)  [unwired: 1 out]
        n159 = Build Path(base path=w189, name or relative path="runnumber.txt") -> (appended path=w187:path)
        n160 = Open/Create/Replace File(file path (use dialog)=w187, operation (0:open)=T4."replace") -> (refnum out=w185:refnum<file>)  [unwired: 4 in, 2 out]
        n161 = Write to Text File(file (use dialog)=w185, text=w183) -> ()  [unwired: 2 in, 3 out]
      }
    }
  }
  n162 = while {
    tunnel: w29 -> [w271]
    shift-right: [w265] -> _
    shift-left: _ -> [w264]
    shift-right: [w263] -> _
    shift-left: _ -> [w261]
    shift-right: [w262] -> _
    shift-left: _ -> [w260]
    shift-right: [w257] -> _
    shift-left: 0 -> [w258]
    shift-right: [w256] -> _
    shift-left: _ -> [w255]
    shift-right: [w254] -> _
    shift-left: _ -> [w253]
    tunnel: w5 -> [w252]
    tunnel: w1 -> [w251]
    stop <- w259 stop-if-true
    # "cam"
    n163 = Preview Queue Element(queue=w271, timeout in ms (-1)=w258) -> (queue out=w270:refnum<queue>, element=w269:string)  [unwired: 1 in, 2 out]
    n164 = Match Pattern(string=w269, regular expression=":") -> (before substring=w266:string, after substring=w267:string)  [unwired: 1 in, 2 out]
    n165 = case shown="\"idle\", Default" w266 {
      tunnel: w270 -> [w279 w307 w335 w375 w385 _ w415 w425 w449]
      tunnel: w267 -> [_ _ w341 _ _ _ _ w428 _]
      tunnel: [w273 w296 w332 w374 w383 w388 w413 w437 w447] -> w265
      tunnel: w264 -> [_ _ w338 w374 w383 w388 w413 w437 w447]
      tunnel: [w278 w308 w333 u64 0 ("Hout") w382 w402 w412 w436 w446] -> w263
      tunnel: [w280 w309 w334 w371 w381 w405 w414 w438 w445] -> w262
      tunnel: w261 -> [_ w311 w337 w373 w382 w392 w417 w424 w446]
      tunnel: w260 -> [_ w310 w336 _ w381 w391 w416 w439 w445]
      tunnel: [_ _ _ _ TRUE _ _ _ _] -> w259
      tunnel: [_ _ _ _ _ _ _ _ -1] -> w257
      tunnel: [w272 w293 _ _ _ w401 _ _ _] -> w256
      tunnel: w255 -> [w272 w293 _ _ _ w400 _ _ _]
      tunnel: [w273 w295 w331 w369 w380 w396 w410 w431 w444] -> w254
      tunnel: w253 -> [_ w295 w331 w369 w380 w396 _ w431 w444]
      tunnel: w252 -> [_ _ w329 _ _ _ _ w435 _]
      tunnel: w251 -> [_ _ _ _ _ _ _ w423 _]
      frame "init" {
        w273 = u16[][] []
        n166 = flat-sequence {
          tunnel: [w282] -> w277
          tunnel: [w283] -> w276
          tunnel: [w291] -> w278
          tunnel: [w292] -> w280
          tunnel: w277 -> [w292]
          tunnel: w276 -> [w291]
          frame #0 {
            n167 = local write "cam_con?"(FALSE ("cam_con?")) -> ()
          }
          frame #1 {
            n168 = call "SCInitBoard.vi"("boardnr"="cam_boardnr") -> ("Hout"=w286:u32, "error out"=w287:errorcluster)  [unwired: 1 in, 1 out]
            n169 = call "SCSetupCamera.vi"("Handle"=w286, "error in (no error)"=w287) -> ("Hout"=w288:u64, "error out"=w289:errorcluster)  [unwired: 1 out]
            n170 = call "SCStopCOC.vi"("error in (no error)"=w289, "Stop mode"=0, "Handle"=w288) -> ("error out"=w282:errorcluster, "Hout"=w283:u64)
          }
          frame #2 {
            n171 = local write "cam_con?"(TRUE ("cam_con?")) -> ()
          }
        }
        n172 = Dequeue Element(queue=w279) -> (queue out=w275:refnum<queue>)  [unwired: 2 in, 3 out]
        n173 = Enqueue Element At Opposite End(queue=w275, element="set") -> ()  [unwired: 2 in, 3 out]
      }
      frame "set" {
        w306 = u32 1 ("Operating mode\nHP & QE / HS & DiCam Pro")
        n174 = Dequeue Element(queue=w307) -> ()  [unwired: 2 in, 4 out]
        n175 = Bundle By Name(cluster=cluster{"Delay":dbl, "Exposure ":dbl} {"Delay"=0.0, "Exposure "=0.0} ("Delay and exposure"), "Exposure"="exposure [ms]") -> (w303:cluster{"Delay":dbl, "Exposure ":dbl})
        n176 = call "SCStopCOC.vi"("error in (no error)"=w310, "Stop mode"=0, "Handle"=w311) -> ("error out"=w326:errorcluster, "Hout"=w325:u64)
        n177 = Bundle By Name(cluster=T5 {"Camera type"=0, "Operating mode\nHP & QE / HS & DiCam Pro "=0, "Frame trigger \n(High Performance and QE only)"=0, "Sequence trigger"=0, "Low Light\n(QE only)"=FALSE, "Gain"=FALSE, "Horzontal\nbinning"=0, "Vertical\nbinning "=0, "ROI Left"=1, "ROI Right"=20, "ROI Top"=1, "ROI Bottom"=15} ("Camera controls"), "Operating mode\nHP & QE / HS & DiCam Pro"=w306, "Horzontal\nbinning"="binning", "Vertical\nbinning"="binning", "ROI Left"="ROI Left", "ROI Right"="ROI Right", "ROI Top"="ROI Top", "ROI Bottom"="ROI Bottom", "Gain"="gain") -> (w321:T5)
        n178 = call "New delay and exposure forma.vi"("Operating mode\nHP & QE / HS & DiCam Pro"=w306, "Delay and exposure"=w303) -> ("Output table"=w322:string)  [unwired: 3 in]
        n179 = call "SCSetCoC.vi"("error in (no error)"=w326, "Delay and exposure table"=w322, "Camera controls"=w321, "Handle"=w325) -> ("error out"=w314:errorcluster, "Hout"=w313:u64)  [unwired: 1 out]
        n180 = call "SCGetImageSize.vi"("Handle"=w313, "error in (no error)"=w314) -> ("Hout"=w312:u64, "error out"=w294:errorcluster, "Horizontal size"=w300:i32, "Vertical size"=w299:i32)  [unwired: 2 out]
        n181 = Greater?(x=w300, y=w299) -> (0:w301:bool)
        n182 = Initialize Array(u16 0 ("dimension size"), w299, w300) -> (w296:u16[][])
        n183 = call "SCRun.vi"("error in (no error)"=w294, "Run mode"=0, "Handle"=w312) -> ("error out"=w309:errorcluster, "Hout"=w308:u64)  [unwired: 1 out]
        n184 = Select(t=w300, s=w301, f=w299) -> (s? t:f=w298:i32)
        n185 = property on="Intensity Graph" class="IntGraph (strict)"("XScale.Maximum"=w298, "YScale.Maximum"=w298) -> ()  [unwired: 2 in, 2 out]
      }
      frame "burst" {
        n186 = Match Pattern(string=w341, regular expression=":") -> (before substring=w340:string, after substring=w339:string)  [unwired: 1 in, 2 out]
        n187 = Dequeue Element(queue=w335) -> ()  [unwired: 2 in, 4 out]
        n188 = Decimal String To Number(string=w340) -> (number=w330:i32)  [unwired: 2 in, 1 out]
        n189 = String To Path(string=w339) -> (path=w327:path)
        n190 = for {
          N: w330 -> [_]
          tunnel: w338 -> [w346]
          tunnel: w337 -> [w347]
          tunnel: w331 -> [w364]
          tunnel: [w344] -> w333
          shift-right: [w343] -> w334
          shift-left: w336 -> [w348]
          tunnel: [w346] -> w332
          tunnel: w329 -> [w362]
          tunnel: 100000 ("x") -> [w355]
          tunnel: w327 -> [w354]
          i -> [w349]
          n191 = local read "cam_dark?"() -> (w363:bool)
          n192 = Add(x=w355, y=w349) -> (x+y=w359:i32)
          n193 = call "grabimg.vi"("array in"=w346, "error in"=w348, "Hin"=w347) -> ("error out"=w343:errorcluster, "imgdata"=w345:dbl[][], "Hout"=w344:u64)  [unwired: 6 in]
          n194 = Number To Decimal String(number=w359) -> (decimal integer string=w358:string)  [unwired: 1 in]
          n195 = String Subset(string=w358, offset (0)=1) -> (substring=w356:string)  [unwired: 1 in]
          n196 = case shown="True" w363 {
            tunnel: w345 -> [w365 w368]
            tunnel: w364 -> [_ w367]
            tunnel: [w365 w366] -> w350
            frame False {
            }
            frame True {
              n197 = Subtract(x=w368, y=w367) -> (x-y=w366:dbl[][])
            }
          }
          n198 = Build Path(base path=w354, name or relative path=w356) -> (appended path=w353:path)
          n199 = Path To String(path=w353) -> (string=w352:string)
          n200 = local write "Intensity Graph"(w350) -> ()
          n201 = Concatenate Strings("save:" ("string"), w352) -> (w351:string)
          n202 = Bundle(w351, "imgdata"=w350) -> (w361:cluster{string, "imgdata":dbl[][]})  [unwired: 1 in]
          n203 = Enqueue Element(queue=w362, element=w361) -> ()  [unwired: 2 in, 3 out]
          "cam_burst_progress" <- w349
        }
        n204 = property on="cam_burst_progress" class="Slide (strict)"("Scale.Maximum"=w330) -> ()  [unwired: 2 in, 2 out]
      }
      frame "release" {
        n205 = Dequeue Element(queue=w375) -> ()  [unwired: 2 in, 4 out]
        n206 = flat-sequence {
          tunnel: w373 -> [w377]
          tunnel: [w376] -> w370
          tunnel: [w379] -> w371
          tunnel: w370 -> [w379]
          frame #0 {
            n207 = call "SCCloseBoard.vi"("Handle"=w377) -> ("error out"=w376:errorcluster)  [unwired: 1 in, 2 out]
          }
          frame #1 {
            n208 = local write "cam_con?"(FALSE ("cam_con?")) -> ()
          }
        }
      }
      frame "close" {
        n209 = Release Queue(queue=w385) -> ()  [unwired: 2 in, 3 out]
      }
      frame "idle", Default {
        n210 = local read "cam_avg"() -> (w387:u32)
        n211 = call "grabimg.vi"("array in"=w388, "error in"=w391, "avg"=w387, "Hin"=w392) -> ("error out"=w389:errorcluster, "imgdata"=w386:dbl[][], "Hout"=w390:u64)  [unwired: 5 in]
        n212 = call "SCGetStatus.vi"("Handle"=w390, "error in (no error)"=w389) -> ("Hout"=w402:u64, "Electronics temperature"=→"electronics temp [°C]":i32, "CCD temperature"=→"CCD temp [°C]":i32, "error out"=w405:errorcluster)  [unwired: 2 out]
        n213 = case shown="False" "cam_dark?" {
          tunnel: w396 -> [_ w409]
          tunnel: [w406 w408] -> w394
          tunnel: w386 -> [w406 w407]
          frame False {
          }
          frame True {
            n214 = Subtract(x=w407, y=w409) -> (x-y=w408:dbl[][])
          }
        }
        "Intensity Graph" <- w394
        n215 = call <vilib>:"High Resolution Relative Seconds.vi"() -> ("relative seconds"=w401:dbl)
        n216 = Array Max & Min(array=w394) -> (max value=→"max value":dbl)  [unwired: 3 out]
        n217 = Add Array Elements(numeric array=w394) -> (sum=→"sum":dbl)
        n218 = Subtract(x=w401, y=w400) -> (x-y=w399:dbl)
        n219 = Reciprocal(x=w399) -> (1/x=→"cam_fps":dbl)
      }
      frame "dark" {
        n220 = Dequeue Element(queue=w415) -> ()  [unwired: 2 in, 4 out]
        n221 = call "grabimg.vi"("array in"=w413, "error in"=w416, "avg"="cam_dark#", "Hin"=w417) -> ("error out"=w414:errorcluster, "imgdata"=w410:dbl[][], "Hout"=w412:u64)  [unwired: 5 in]
      }
      frame "snap" {
        n222 = Dequeue Element(queue=w425) -> ()  [unwired: 2 in, 4 out]
        n223 = Match Pattern(string=w428, regular expression=":") -> (before substring=w427:string, after substring=w426:string)  [unwired: 1 in, 2 out]
        n224 = Decimal String To Number(string=w427) -> (number=w419:i32)  [unwired: 2 in, 1 out]
        n225 = local read "cam_dark?"() -> (w430:bool)
        n226 = call "grabimg.vi"("array in"=w437, "error in"=w439, "avg"=w419, "Hin"=w424) -> ("error out"=w438:errorcluster, "imgdata"=w420:dbl[][], "Hout"=w436:u64)  [unwired: 5 in]
        n227 = Concatenate Strings("save:" ("string"), w426) -> (w434:string)
        n228 = case shown="True" w430 {
          tunnel: [w440 w441] -> w418
          tunnel: w420 -> [w440 w443]
          tunnel: w431 -> [_ w442]
          frame False {
          }
          frame True {
            n229 = Subtract(x=w443, y=w442) -> (x-y=w441:dbl[][])
          }
        }
        n230 = Bundle(w434, "imgdata"=w418) -> (w433:cluster{string, "imgdata":dbl[][]})  [unwired: 1 in]
        n231 = Enqueue Element(queue=w435, element=w433) -> (error out=w421:errorcluster)  [unwired: 2 in, 2 out]
        n232 = Enqueue Element(queue=w423, element="done", error in (no error)=w421) -> ()  [unwired: 1 in, 3 out]
      }
      frame "suspend" {
        n233 = Dequeue Element(queue=w449) -> ()  [unwired: 2 in, 4 out]
      }
    }
    "error out" <- w262
  }
  n234 = while {
    tunnel: w18 -> [w458]
    shift-right: [w456] -> _
    shift-left: _ -> [w454]
    shift-right: [w455] -> _
    shift-left: _ -> [w453]
    shift-right: [w451] -> _
    shift-left: 0 -> [w452]
    tunnel: w1 -> [w450]
    stop <- w457 stop-if-true
    # "ESP"
    n235 = Preview Queue Element(queue=w458, timeout in ms (-1)=w452) -> (queue out=w461:refnum<queue>, element=w462:string)  [unwired: 1 in, 2 out]
    n236 = Match Pattern(string=w462, regular expression=":") -> (before substring=w460:string, after substring=w459:string)  [unwired: 1 in, 2 out]
    n237 = case shown="\"abs\"" w460 {
      tunnel: w461 -> [_ w476 w494 w528 w529 w536 w541]
      tunnel: w459 -> [_ w481 w501 _ _ _ _]
      tunnel: [_ _ _ _ _ TRUE _] -> w457
      tunnel: [w465 w483 w495 w526 refnum<visa-resource-name> refnum ("VISA resource name out") w533 w540] -> w456
      tunnel: [w464 w484 w493 w525 w531 w534 w539] -> w455
      tunnel: w454 -> [w472 w486 w499 w526 w532 w533 _]
      tunnel: w453 -> [w471 w485 w500 w525 _ w534 _]
      tunnel: [_ _ _ -1 _ _ _] -> w451
      tunnel: w450 -> [_ _ w492 _ _ _ _]
      frame "idle", Default {
        n238 = local read "ESP Axis"() -> (w466:i32)
        n239 = local read "ESP_t0"() -> (w475:dbl)
        n240 = call "Read Actual Position.vi"("error in (no error)"=w471, "Axis (1)"=w466, "VISA resource name"=w472) -> ("error out"=w469:errorcluster, "Position (units)"=w470:dbl, "VISA resource name out"=w468:refnum<visa-resource-name>)  [unwired: 2 in]
        "ESP_pos" <- w470
        n241 = call "Get Axis Motion Status.vi"("error in (no error)"=w469, "Axis (1)"=w466, "VISA resource name"=w468) -> ("error out"=w464:errorcluster, "Motion Done"=→"Motion Done":bool, "VISA resource name out"=w465:refnum<visa-resource-name>)  [unwired: 2 in]
        n242 = call "mm2time.vi"("fs?"=TRUE, "Offset (mm)"=w475, "distance (mm)"=w470) -> ("time in fs/ps seconds"=→"ESP_delay":dbl)
      }
      frame "rel" {
        n243 = Match Pattern(string=w481, regular expression=":") -> (before substring=w480:string, after substring=w479:string)  [unwired: 1 in, 2 out]
        n244 = Dequeue Element(queue=w476) -> ()  [unwired: 2 in, 4 out]
        n245 = Decimal String To Number(string=w480) -> (number=w478:i32)  [unwired: 2 in, 1 out]
        n246 = Fract/Exp String To Number(string=w479) -> (number=w477:dbl)  [unwired: 3 in, 1 out]
        n247 = call "Move Relative.vi"("error in (no error)"=w485, "Position (0 units)"=w477, "Axis (1)"=w478, "VISA resource name"=w486) -> ("error out"=w484:errorcluster, "VISA resource name out"=w483:refnum<visa-resource-name>)  [unwired: 2 in]
      }
      frame "abs" {
        n248 = Match Pattern(string=w501, regular expression=":") -> (before substring=w502:string, after substring=w490:string)  [unwired: 1 in, 2 out]
        n249 = Dequeue Element(queue=w494) -> ()  [unwired: 2 in, 4 out]
        n250 = Match Pattern(string=w490, regular expression=":") -> (before substring=w489:string, after substring=w488:string)  [unwired: 1 in, 2 out]
        n251 = Decimal String To Number(string=w502) -> (number=w498:i32)  [unwired: 2 in, 1 out]
        n252 = Fract/Exp String To Number(string=w489) -> (number=w487:dbl)  [unwired: 3 in, 1 out]
        n253 = call "Move Absolute.vi"("error in (no error)"=w500, "Position (0 units)"=w487, "Axis (1)"=w498, "VISA resource name"=w499) -> ("error out"=w496:errorcluster, "VISA resource name out"=w497:refnum<visa-resource-name>)  [unwired: 2 in]
        n254 = case shown="\"wait\"" w488 {
          tunnel: w498 -> [_ w510]
          tunnel: w497 -> [w505 w515]
          tunnel: w496 -> [w504 w514]
          tunnel: [w505 w507] -> w495
          tunnel: [w504 w513] -> w493
          tunnel: w492 -> [_ w512]
          frame "", Default {
          }
          frame "wait" {
            n255 = while {
              tunnel: w510 -> [w524]
              shift-right: [w521] -> w509
              shift-left: w515 -> [w523]
              shift-right: [w520] -> w508
              shift-left: w514 -> [w522]
              stop <- w519 stop-if-true
              n256 = call "Get Axis Motion Status.vi"("error in (no error)"=w522, "Axis (1)"=w524, "VISA resource name"=w523) -> ("error out"=w520:errorcluster, "Motion Done"=w519:bool, "VISA resource name out"=w521:refnum<visa-resource-name>)  [unwired: 2 in]
            }
            n257 = flat-sequence {
              tunnel: w509 -> [w518]
              tunnel: w508 -> [w517]
              tunnel: [w518] -> w507
              tunnel: [w517] -> w506
              frame #0 {
                n258 = Wait (ms)(milliseconds to wait=u32 1000) -> ()  [unwired: 1 out]
              }
            }
            n259 = Enqueue Element(queue=w512, element="done", error in (no error)=w506) -> (error out=w513:errorcluster)  [unwired: 1 in, 2 out]
          }
        }
      }
      frame "suspend" {
        n260 = Dequeue Element(queue=w528) -> ()  [unwired: 2 in, 4 out]
      }
      frame "release" {
        n261 = Dequeue Element(queue=w529) -> ()  [unwired: 2 in, 4 out]
        n262 = call "Close.vi"("VISA resource name"=w532) -> ("error out"=w531:errorcluster)  [unwired: 10 in]
      }
      frame "close" {
        n263 = Release Queue(queue=w536) -> ()  [unwired: 2 in, 3 out]
      }
      frame "init" {
        n264 = Dequeue Element(queue=w541) -> ()  [unwired: 2 in, 4 out]
        n265 = flat-sequence {
          tunnel: [w544] -> w538
          tunnel: [w543] -> w537
          tunnel: [w548] -> w539
          tunnel: [w549] -> w540
          tunnel: w538 -> [w549]
          tunnel: w537 -> [w548]
          frame #0 {
            n266 = local write "ESP_con?"(FALSE ("ESP_con?")) -> ()
          }
          frame #1 {
            n267 = call "Initialize.vi"("VISA resource name"="ESP301 VISA", "Serial Link (RS232)"=enum16{"RS232", "USB"}."USB") -> ("VISA resource name out"=w544:refnum<visa-resource-name>, "error out"=w543:errorcluster)  [unwired: 7 in]
          }
          frame #2 {
            n268 = local write "ESP_con?"(TRUE ("ESP_con?")) -> ()
          }
        }
      }
    }
  }
  n269 = while {
    tunnel: w17 -> [w557]
    shift-right: [w555] -> _
    shift-left: _ -> [w553]
    shift-right: [w554] -> _
    shift-left: _ -> [w552]
    shift-right: [w550] -> _
    shift-left: 0 -> [w551]
    stop <- w556 stop-if-true
    # "manip"
    n270 = Preview Queue Element(queue=w557, timeout in ms (-1)=w551) -> (queue out=w560:refnum<queue>, element=w561:string)  [unwired: 1 in, 2 out]
    n271 = Match Pattern(string=w561, regular expression=":") -> (before substring=w559:string, after substring=w558:string)  [unwired: 1 in, 2 out]
    n272 = case shown="\"idle\", Default" w559 {
      tunnel: w560 -> [_ _ w578 w582 w591 w602]
      tunnel: w558 -> [_ _ _ _ _ _]
      tunnel: [_ _ _ _ TRUE _] -> w556
      tunnel: [w564 w566 w580 refnum<k5> refnum ("gateway_connection out") w589 w593] -> w555
      tunnel: [w563 w565 w579 w584 w588 w592] -> w554
      tunnel: w553 -> [w564 w566 w580 w586 w589 _]
      tunnel: w552 -> [w563 w565 w579 _ w588 _]
      tunnel: [_ _ -1 _ _ _] -> w550
      frame "idle", Default {
      }
      frame "relative" {
        n273 = disable-structure shown="Disabled" {
          frame Disabled {
            n274 = case shown="True" FALSE {
              tunnel: [_ w576] -> w568
              frame False {
              }
              frame True {
                n275 = call "sp_manip_get_axis_status.vi"("gateway_connection"=w576) -> ("error out"=w571:errorcluster, "axis_out"=w575:T6, "gateway_connection out"=w569:refnum<k5>)  [unwired: 6 in, 2 out]
                n276 = Index Array(array=w575) -> (element=w574:T7, index=w577:i32)
                n277 = Unbundle By Name(w574) -> ("Axis_Name"=w570:string)  [unwired: 1 out]
                n278 = Build Array(w570) -> (w573:string[])
                n279 = Build Array() -> (w572:void[])  [unwired: 1 in]
                n280 = call "sp_manip_start_move.vi"("error in"=w571, "target positions"=w572, "axis names"=w573, "gateway_connection"=w569) -> ()  [unwired: 4 in, 4 out]
              }
            }
          }
          frame Enabled {
          }
        }
      }
      frame "suspend" {
        n281 = Dequeue Element(queue=w578) -> ()  [unwired: 2 in, 4 out]
      }
      frame "release" {
        n282 = Dequeue Element(queue=w582) -> ()  [unwired: 2 in, 4 out]
        n283 = call "sp_manip_disconnect.vi"("gateway_connection"=w586) -> ("error out"=w585:errorcluster, "gateway_connection_out"=w587:refnum<k5>)  [unwired: 7 in, 2 out]
        n284 = call "tcp_gateway_close_connection.vi"("error in"=w585, "server_connection"=w587) -> ("error out"=w584:errorcluster)  [unwired: 5 in]
      }
      frame "close" {
        n285 = Release Queue(queue=w591) -> ()  [unwired: 2 in, 3 out]
      }
      frame "init" {
        n286 = Dequeue Element(queue=w602) -> ()  [unwired: 2 in, 4 out]
        n287 = call "tcp_gateway_open_connection.vi"() -> ("gateway_connection"=w597:refnum<k5>, "error out"=w596:errorcluster)  [unwired: 5 in, 3 out]
        n288 = call "sp_manip_connect.vi"("error in"=w596, "gateway_connection"=w597) -> ("error out"=w592:errorcluster, "axis_out"=w595:T6, "gateway_connection out"=w593:refnum<k5>)  [unwired: 5 in, 2 out]
        n289 = for {
          tunnel: w595 -> [w605] mode=indexing
          tunnel: [w604] -> w600 mode=indexing
          tunnel: [w603] -> w601 mode=indexing
          n290 = Unbundle By Name(w605) -> ("Axis_Name"=w604:string, "Axis_Position"=w603:dbl)
        }
        "names" <- w600
        "pos" <- w601
        n291 = control-ref of="meas_axis"() -> (w594:refnum<vi>)
        n292 = local write "dest"(w601) -> ()
        n293 = Build Array (concatenate)(w600, "XY") -> (w598:string[])
        n294 = property on="Property Node" class="CmbBox"(reference=w594, "Strings[]"=w598) -> ()  [unwired: 1 in, 2 out]
      }
    }
  }
  n295 = while {
    tunnel: w16 -> [w616]
    shift-right: [w613] -> _
    shift-left: 0 -> [w614]
    shift-right: [w612] -> _
    shift-left: _ -> [w611]
    shift-right: [w610] -> _
    shift-left: _ -> [w609]
    shift-right: [w608] -> _
    shift-left: u32 0 ("pHandle") -> [w607]
    tunnel: string[] ["Kinetic Energy", "Pass Energy", "Coil Current", "Work Function", "Detector Voltage", "Screen Voltage", "Conversion Voltage", "Focus Displacement 1", "Focus Displacement 2"] -> [w606]
    stop <- w615 stop-if-true
    # "phoib"
    n296 = Preview Queue Element(queue=w616, timeout in ms (-1)=w614) -> (queue out=w619:refnum<queue>, element=w620:string)  [unwired: 1 in, 2 out]
    n297 = Match Pattern(string=w620, regular expression=":") -> (before substring=w618:string, after substring=w617:string)  [unwired: 1 in, 2 out]
    n298 = case shown="\"init\"" w618 {
      tunnel: w619 -> [_ w673 w689 w705 w719 w723 w729]
      tunnel: w617 -> [_ _ _ _ _ _ _]
      tunnel: [_ _ _ _ TRUE _ _] -> w615
      tunnel: [_ _ _ _ _ -1 _] -> w613
      tunnel: [w630 w675 w692 w703 w717 w722 w726] -> w612
      tunnel: w611 -> [w641 w664 w694 w704 w717 w722 _]
      tunnel: [w629 w674 w691 w702 w715 w720 w725] -> w610
      tunnel: w609 -> [w639 w663 w693 _ w715 w720 _]
      tunnel: [w627 w661 w690 w701 w716 w721 w728] -> w608
      tunnel: w607 -> [w627 w661 w690 w700 w716 w721 _]
      tunnel: w606 -> [w628 w654 _ _ _ _ _]
      frame "idle", Default {
        n299 = call "SL2_AD_DLL_Phoibos_GetDeviceState.vi"("dll_path"=w641, "pHandle_in"=w627, "dev_type"=DEF_dev_type."devA (analyzer)", "error in"=w639) -> ("path out"=w626:path, "state"=→"state":T3, "error out"=w625:errorcluster)  [unwired: 2 in]
        n300 = for {
          tunnel: w627 -> [w648]
          tunnel: w628 -> [w646] mode=indexing
          tunnel: [w645] -> w638 mode=indexing
          tunnel: [w644] -> w630
          shift-right: [w643] -> w629
          shift-left: w625 -> [w647]
          tunnel: w626 -> [w642]
          n301 = call "SL2_AD_DLL_Phoibos_GetVoltage.vi"("error in"=w647, "voltage_name"=w646, "pHandle"=w648, "dll path in"=w642) -> ("error out"=w643:errorcluster, "value"=w645:dbl, "dll path out"=w644:path)  [unwired: 3 in]
        }
        n302 = Index Array(array=w638) -> (element #1=→"phoib_I_1":dbl, element #2=→"phoib_I_2":dbl, element #3=→"phoib_I_3":dbl, element #4=→"phoib_I_4":dbl, element #5=→"phoib_I_5":dbl, element #6=→"phoib_I_6":dbl, element #7=→"phoib_I_7":dbl, element #8=→"phoib_I_8":dbl, element #9=→"phoib_I_9":dbl)  [unwired: 9 in]
      }
      frame "set" {
        n303 = Dequeue Element(queue=w673) -> ()  [unwired: 2 in, 4 out]
        n304 = Multiply(x="VoltageRange", y=13) -> (x*y=w670:i32)
        n305 = Add(x="Mode", y=w670) -> (x+y=w667:i32)
        n306 = Index Array(array=u32[] [251749632, 251749633, 251749634, 251749635, 251749636, 251749637, 251749638, 251749639, 251749640, 251749641, 251749642, 251749643, 251749644, 251749645, 251749646, 251749647, 251749648, 251749649, 251749650, 251749651, 251749652, 251749653, 251749654, 251749655, 251749656, 251749657, 251749658, 251749659, 251749660, 251749661, 251749662, 251749663, 251749664, 251749665, 251749666, 251749667, 251749668, 251749669, 251749670, 251749671, 251749672, 251749673, 251749674, 251749675, 251749676, 251749677, 251749678, 251749679, 251749680, 251749681, 251749682, 251749683, 251749684, 251749685, 251749686, 251749687, 251749688, 251749689, 251749690, 251749691, 251749692, 251749693, 251749694, 251749695, 251749696] ("modeIDs"), index=w667) -> (element=w665:u32)
        n307 = Build Array("phoib_I_1s", "phoib_I_2s", "phoib_I_3s", "phoib_I_4s", "phoib_I_5s", "phoib_I_6s", "phoib_I_7s", "phoib_I_8s", "phoib_I_9s") -> (w653:dbl[])
        n308 = call "SL2_AD_DLL_Phoibos_SetDeviceMode.vi"("pHandle"=w661, "error in"=w663, "value"=w665, "dev_type"=DEF_dev_type."devA (analyzer)", "dll path in"=w664) -> ("error out"=w652:errorcluster, "dll path out"=w662:path)  [unwired: 4 in]
        n309 = for {
          tunnel: w661 -> [w681]
          shift-right: [w688] -> w675
          shift-left: w662 -> [w685]
          tunnel: w654 -> [w680] mode=indexing
          tunnel: w653 -> [w679] mode=indexing
          shift-right: [w687] -> w674
          shift-left: w652 -> [w683]
          n310 = call "SL2_AD_DLL_Phoibos_GetVoltageRange.vi"("error in"=w683, "voltage_name"=w680, "pHandle"=w681, "dll path in"=w685) -> ("error out"=w682:errorcluster, "min"=w677:dbl, "max"=w678:dbl, "dll path out"=w684:path)  [unwired: 2 in]
          n311 = In Range and Coerce(upper limit=w678, x=w679, lower limit=w677) -> (coerced(x)=w676:dbl)  [unwired: 1 out]
          n312 = call "SL2_AD_DLL_Phoibos_SetVoltage.vi"("commit"=TRUE, "pHandle"=w681, "error in"=w682, "value"=w676, "voltageName"=w680, "dll path in"=w684) -> ("error out"=w687:errorcluster, "dll path out"=w688:path)  [unwired: 3 in]
        }
      }
      frame "standby" {
        w695 = T3 0 items=["Off"=-1, "Standby"=0, "On"=1] ("state")
        n313 = Dequeue Element(queue=w689) -> ()  [unwired: 2 in, 4 out]
        n314 = call "SL2_AD_DLL_Phoibos_SetDeviceState.vi"("pHandle_in"=w690, "error in"=w693, "state"=w695, "dev_type"=DEF_dev_type."devA (analyzer)", "dll_path"=w694) -> ("error out"=w691:errorcluster, "path out"=w692:path)  [unwired: 2 in]
      }
      frame "release" {
        n315 = Dequeue Element(queue=w705) -> ()  [unwired: 2 in, 4 out]
        n316 = flat-sequence {
          tunnel: w704 -> [w706]
          tunnel: w700 -> [w707]
          tunnel: [w710] -> w699
          tunnel: [w709] -> w698
          tunnel: [u32 0] -> w697
          tunnel: [w712] -> w701
          tunnel: [w713] -> w702
          tunnel: [w714] -> w703
          tunnel: w699 -> [w714]
          tunnel: w698 -> [w713]
          tunnel: w697 -> [w712]
          frame #0 {
            n317 = call "SL2_AD_DLL_Phoibos_Shutdown.vi"("pHandle"=w707, "dll path in"=w706) -> ("error out"=w709:errorcluster, "dll path out"=w710:path)  [unwired: 4 in]
          }
          frame #1 {
            n318 = local write "phoib_con?"(FALSE ("phoib_con?")) -> ()
          }
        }
      }
      frame "close" {
        n319 = Release Queue(queue=w719) -> ()  [unwired: 2 in, 3 out]
      }
      frame "suspend" {
        n320 = Dequeue Element(queue=w723) -> ()  [unwired: 2 in, 4 out]
      }
      frame "init" {
        n321 = Dequeue Element(queue=w729) -> ()  [unwired: 2 in, 4 out]
        n322 = flat-sequence {
          tunnel: [w736] -> w727
          tunnel: [w732] -> w726
          tunnel: [w731] -> w725
          tunnel: [w744] -> w728
          tunnel: w727 -> [w744]
          frame #0 {
            n323 = local write "phoib_con?"(FALSE ("phoib_con?")) -> ()
          }
          frame #1 {
            w735 = DEF_dev_type."devA (analyzer)" ("dev_type")
            n324 = call "GetSL2AD_VI_dllPath.vi"() -> ("error"=w739:errorcluster, "Path"=w740:path)  [unwired: 9 in, 1 out]
            n325 = call "SL2_AD_DLL_List_Devices.vi"("error in"=w739, "dev_type"=w735, "dll path in"=w740) -> ("error out"=w733:errorcluster, "devices"=w742:string[], "dll path out"=w734:path)  [unwired: 2 in]
            n326 = Index Array(array=w742) -> (element=w741:string)  [unwired: 1 in]
            n327 = call "SL2_AD_DLL_Phoibos_Initialize.vi"("error in"=w733, "analyzerId"=w741, "dll_path"=w734) -> ("error out"=w737:errorcluster, "pHandle"=w736:u32, "path out"=w738:path)  [unwired: 2 in]
            n328 = call "SL2_AD_DLL_Phoibos_ListDeviceModes.vi"("dll path in"=w738, "dev_type"=w735, "pHandle"=w736, "error in"=w737) -> ("dll path out"=w732:path, "error out"=w731:errorcluster)  [unwired: 1 in, 2 out]
          }
          frame #2 {
            n329 = local write "phoib_con?"(TRUE ("phoib_con?")) -> ()
          }
        }
      }
    }
    "error out 2" <- w610
  }
